vi "Find unclipped interval.vi"(4 "Max":dbl=3.45, 6 "Min":dbl=-3.45, 10 "Start":i32, 11 "Data":dbl[](array[numeric])) -> ()   [LabVIEW 2015]
panel:
  out "fractional index or x 2":dbl
  out "fractional index or x":dbl
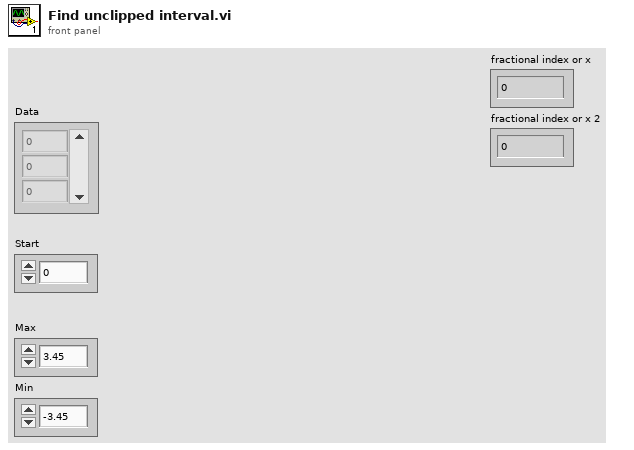
[diagram p1: front panel]
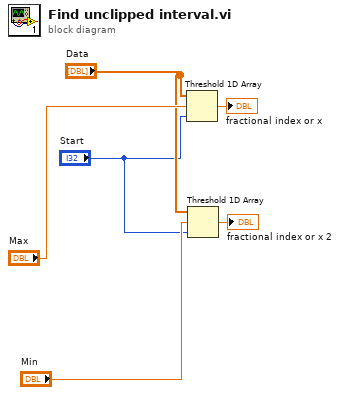
[diagram p0: block diagram]
diagram:
  n1 = Threshold 1D Array(1:"Start", 2:"Max", 3:"Data") -> (0:→"fractional index or x":dbl)
  n2 = Threshold 1D Array(1:"Start", 2:"Min", 3:"Data") -> (0:→"fractional index or x 2":dbl)
